vi "Test_onesetup.vi"() -> ()   [LabVIEW 2015]
uses:
  <vilib>/rvi/Emulation/niFpgaGetClockAttributes.vi
  <vilib>/rvi/Emulation/niFpgaSctlEmulationGetInTimedLoop.vi
  <vilib>/rvi/Emulation/niFpgaEmulationReportErrorSimple.vi
  <vilib>/rvi/eio/common/nirviEmuTemplateMethod_errors.vi
  <vilib>/rvi/interface/RandomDataEmulation/niFpgaRandomDataHandleErrors.vi
  <vilib>/rvi/Emulation/niFpgaCriticalErrorInLSC.vi
  <vilib>/eio/EIONode/EIONode.xnode
  <vilib>/rvi/DataTransferAndStorage/Container/XNode/niFpgaContainer.xnode
  <vilib>/rvi/interface/RandomDataEmulation/nirviRandomDataFpgaReadWriteTemplate.vi
panel:
  in  "stop LED illumination J1":bool
  in  "Low Period (ticks) J1":u32=40000000
  in  "High Period (ticks) J1":u32=40000000
  in  "Apply J1":bool
  out "Tick Count(Ticks) J1":u32 caption="Tick Count(Ticks)"
  in  "Output Enable J1":bool
  in  "FPGA Stop J1":bool
  in  "Half-clock time J1":u32=10
  out "ConnectorB/DIO0, J1":bool=TRUE
  out "Frame Count J1":i16=5
  in  "IRQ Bit (0-31) J1":u8
  in  "Wait Until IRQ Cleared? J1":bool
  out "Timed Out? J1":bool
  out "ConnectorB/AI0 J1":u16=44020
  out "ConnectorB/DIO1 J1":bool
  in  "double number of samples to take per frame J1":u16=1540
  in  "Half-clocks between frames J1":u16=1600
  in  "ConnectorB/AO0 J1":u16
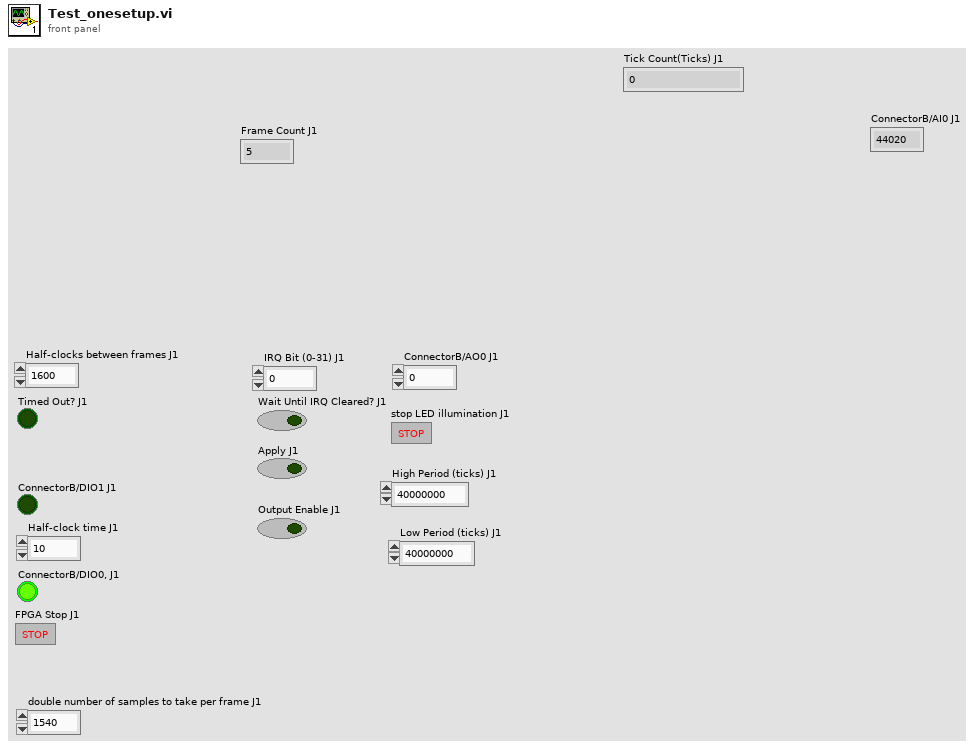
[diagram p1: front panel]
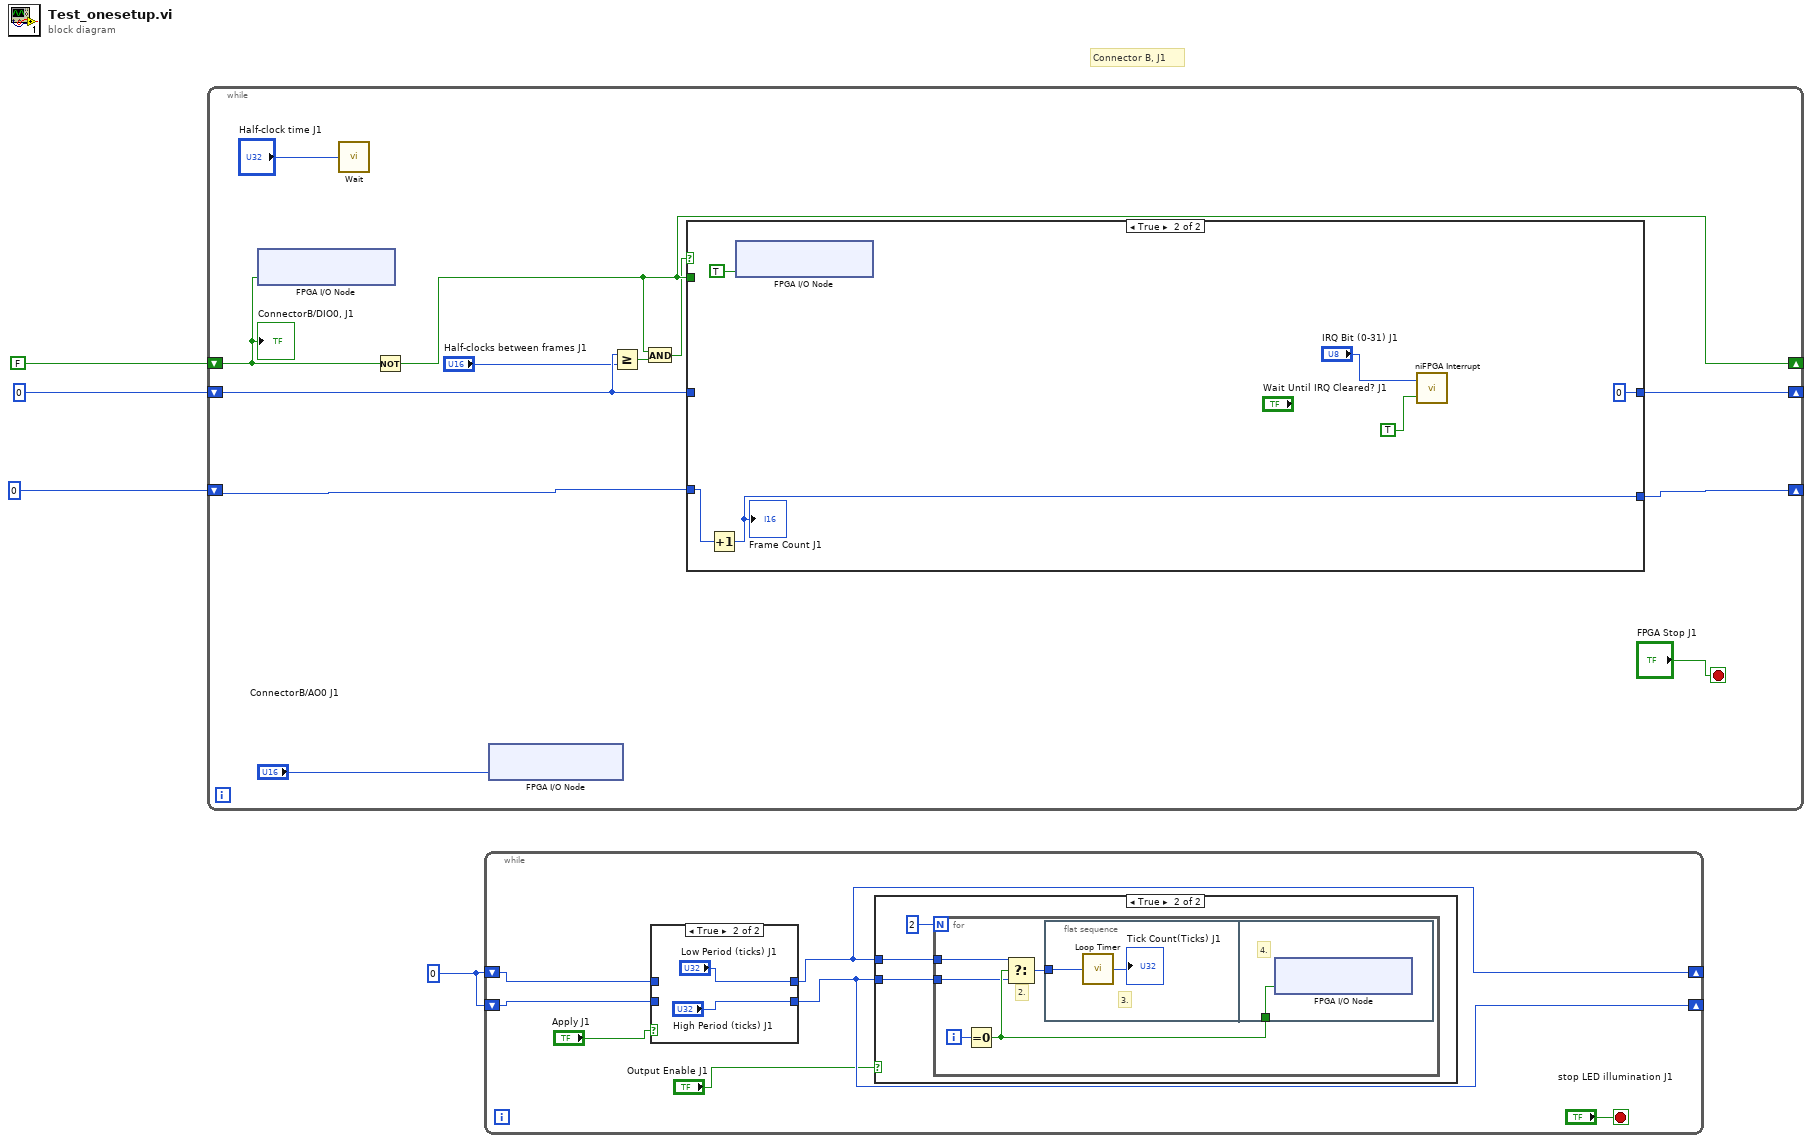
[diagram p0: block diagram]
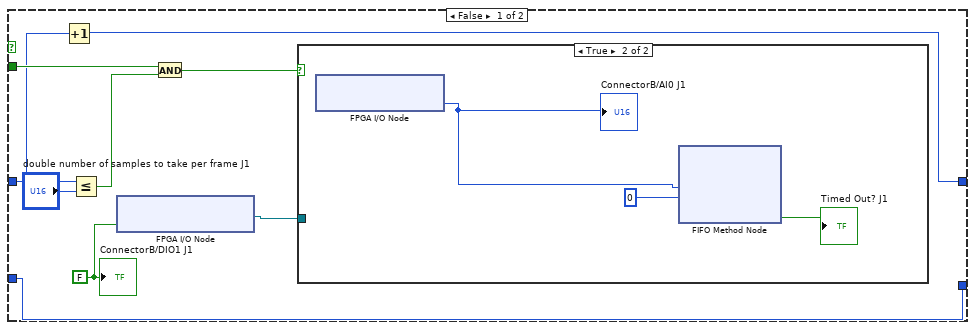
[diagram p4: hidden frame]
diagram:
  w1 = u32 0 ("High Period")
  # "Connector B, J1"
  n1 = while {
    shift-right: [w15] -> _
    shift-left: FALSE ("ConnectorB/DIO0") -> [w16]
    shift-right: [w12] -> _
    shift-left: u16 0 -> [w14]
    shift-right: [w10] -> _
    shift-left: i16 0 -> [w11]
    stop <- "FPGA Stop J1" stop-if-true
    n2 = xnode "FPGA I/O Node"("ConnectorB/DIO0"=w16) -> ()  [unwired: 1 in, 1 out]
    n3 = call "Wait"("Count(uSec)"="Half-clock time J1") -> ()  [unwired: 1 out]
    n4 = Not(x=w16) -> (.not. x?=w15:bool)
    n5 = xnode "FPGA I/O Node"("ConnectorB/AO0"="ConnectorB/AO0 J1") -> ()  [unwired: 1 in, 1 out]
    n6 = Greater Or Equal?(x=w14, y="Half-clocks between frames J1") -> (x >= y?=w8:bool)
    n7 = And(x=w15, y=w8) -> (x .and. y?=w6:bool)
    n8 = case shown="True" w6 {
      tunnel: w14 -> [w20 _]
      tunnel: [w18 u16 0] -> w12
      tunnel: w15 -> [w24 _]
      tunnel: w11 -> [w19 w32]
      tunnel: [w19 w31] -> w10
      frame False {
        w25 = FALSE ("ConnectorB/DIO1")
        n9 = Increment(x=w20) -> (x+1=w18:u16)
        n10 = Less Or Equal?(x=w20, y="double number of samples to take per frame J1") -> (x <= y?=w22:bool)
        n11 = xnode "FPGA I/O Node"("ConnectorB/DIO1"=w25) -> ("FPGA I/O Out"=w21:refnum<k21>)  [unwired: 1 in]
        n12 = And(x=w24, y=w22) -> (x .and. y?=w23:bool)
        n13 = case shown="True" w23 {
          tunnel: w21 -> [_ _]
          frame False {
          }
          frame True {
            n14 = xnode "FPGA I/O Node"() -> ("ConnectorB/AI0"=w28:u16)  [unwired: 1 in, 1 out]
            "ConnectorB/AI0 J1" <- w28
            n15 = xnode ("FIFO Method Node")("Element"=w28, "Timeout"=0) -> ("Timed Out?"=→"Timed Out? J1":bool)  [unwired: 1 in, 1 out]
          }
        }
        "ConnectorB/DIO1 J1" <- w25
      }
      frame True {
        n16 = Increment(x=w32) -> (x+1=w31:i16)
        "Frame Count J1" <- w31
        n17 = xnode "FPGA I/O Node"("ConnectorB/DIO1"=TRUE) -> ()  [unwired: 1 in, 1 out]
        n18 = call <vilib>:"niFPGA Interrupt.vi"("Wait Until Cleared (F)"=TRUE, "IRQ Number (0)"="IRQ Bit (0-31) J1") -> ()  [unwired: 1 in]
      }
    }
    "ConnectorB/DIO0, J1" <- w16
  }
  n19 = while {
    shift-right: [w36] -> _
    shift-left: w1 -> [w40]
    shift-right: [w37] -> _
    shift-left: w1 -> [w39]
    stop <- "stop LED illumination J1" stop-if-true
    n20 = case shown="True" "Apply J1" {
      tunnel: [w54 "Low Period (ticks) J1"] -> w36
      tunnel: [w53 "High Period (ticks) J1"] -> w37
      tunnel: w40 -> [w54 _]
      tunnel: w39 -> [w53 _]
      frame False {
      }
      frame True {
      }
    }
    n21 = case shown="True" "Output Enable J1" {
      tunnel: w36 -> [_ w43]
      tunnel: w37 -> [_ w42]
      frame False {
      }
      frame True {
        n22 = for {
          N: 2 -> [_]
          tunnel: w43 -> [w46]
          tunnel: w42 -> [w45]
          i -> [w48]
          # "2."
          n23 = Equal To 0?(x=w48) -> (x = 0?=w47:bool)
          n24 = Select(t=w46, s=w47, f=w45) -> (s? t:f=w49:u32)
          n25 = flat-sequence {
            tunnel: w49 -> [w51]
            tunnel: w47 -> [w52]
            frame #0 {
              # "3."
              n26 = call "Loop Timer"("Count(Ticks)"=w51) -> ("Tick Count(Ticks)"=→"Tick Count(Ticks) J1":u32)
            }
            frame #1 {
              # "4."
              n27 = xnode "FPGA I/O Node"("ConnectorB/DIO8"=w52) -> ()  [unwired: 1 in, 1 out]
            }
          }
        }
      }
    }
  }
